vi "niRFUtil WFM Remove Frequency Offset - Fine.vi"(0 "Waveform In":T2 {"y" format="%.2f"; "dx" format="%^.2e"; "x0" format="%^.2e"}, 5 "Reference Waveform In":T2 {"y" format="%.2f"; "dx" format="%^.2e"; "x0" format="%^.2e"}, 7 "Filter Phase Estimates":T1=enum."True", 9 "Filter Length (samples)":i32=20) -> (4 "Waveform Out":T2 {"y" format="%.2f"; "dx" format="%^.2e"; "x0" format="%^.2e"}, 6 "Reference Waveform Out":T2 {"y" format="%.2f"; "dx" format="%^.2e"; "x0" format="%^.2e"}, 13 "Offset, Hz":sgl format="%^.2e")   [LabVIEW 2015, in "niRFUtil.lvlib"]
doc: "(c) Copyright 2006, National Instruments, Inc. This VI may not be duplicated, sold, or distributed without written consent from National Instruments."
uses:
  niRFUtil.lvlib
  Includes/niRFUtil INC Complex Waveform.ctl
  Includes/niRFUtil INC Complex Array.ctl
  Includes/niRFUtil INC Filter Phase Estimates.ctl
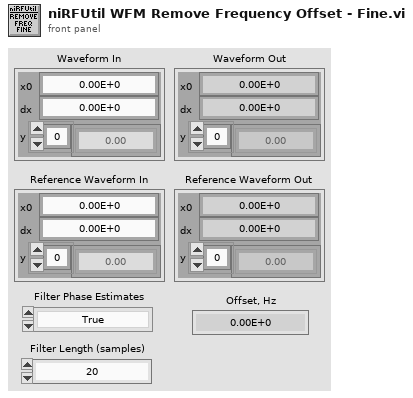
[diagram p1: front panel]
types:
  T1 = typedef "niRFUtil.lvlib/niRFUtil INC Filter Phase Estimates.ctl" = enum16{"False", "True"}
  T2 = typedef "niRFUtil.lvlib/niRFUtil INC Complex Waveform.ctl" = cluster{"x0":dbl, "dx":dbl, "y":T3}
  T3 = typedef "niRFUtil.lvlib/niRFUtil INC Complex Array.ctl" = csg[]
  T4 = typedef "niRFUtil.lvlib/niRFUtil INC Real Array.ctl" = sgl[]
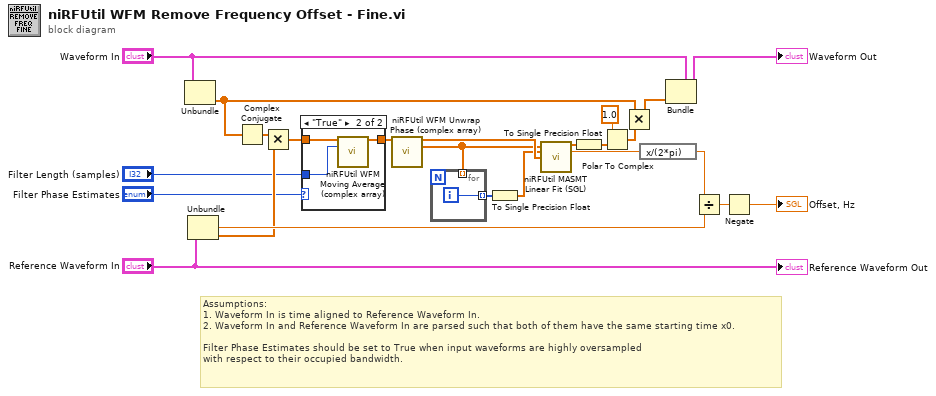
[diagram p0: block diagram]
diagram:
  # "Assumptions:\n1. Waveform In is time aligned to Reference Waveform In.\n2. Waveform In and Reference Waveform In are parsed such that both of them have the same starting time x0.\n\nFilter Phase Estimates should be set to True when input waveforms are highly oversampled\nwith respect to their occupied bandwidth."
  n1 = Unbundle("Waveform In") -> ("y"=w14:T3)  [unwired: 2 out]
  n2 = Unbundle("Reference Waveform In") -> ("dx"=w21:dbl, "y"=w20:T3)  [unwired: 1 out]
  n3 = Complex Conjugate(1:w14) -> (0:w23:T3)
  n4 = Multiply(x=w23, y=w20) -> (x*y=w24:T3)
  n5 = case shown="\"True\"" "Filter Phase Estimates" {
    tunnel: w24 -> [w25 w28]
    tunnel: [w25 w27] -> w4
    tunnel: "Filter Length (samples)" -> [_ w26]
    frame "False" {
    }
    frame "True" {
      n6 = call "niRFUtil WFM Moving Average (complex array).vi"("Array In"=w28, "Averaging Window (samples)"=w26) -> ("Averaged Array Out"=w27:T3)  [unwired: 13 in]
    }
  }
  n7 = call "niRFUtil WFM Unwrap Phase (complex array).vi"("Complex Vectors"=w4) -> ("Magnitude"=w8:T4, "Unwrapped Phase (rad)"=w3:T4)  [unwired: 13 in]
  n8 = for {
    tunnel: [w29] -> w7 mode=indexing
    tunnel: w3 -> [_] mode=indexing
    i -> [w29]
  }
  n9 = To Single Precision Float(number=w7) -> (single precision float=w6:sgl[])
  n10 = call "niRFUtil MASMT Linear Fit (SGL).vi"("Y"=w3, "X"=w6, "Weight"=w8) -> ("Best Linear Fit"=w12:sgl[], "slope"=w17:sgl)  [unwired: 8 in, 3 out]
  n11 = To Single Precision Float(number=w12) -> (single precision float=w5:sgl[])
  n12 = Polar To Complex(1:w5, 2:sgl 1.0) -> (0:w10:csg[])
  n13 = Multiply(x=w14, y=w10) -> (x*y=w13:T3)
  n14 = expression code="x/(2*pi)"(w17) -> (w19:sgl)
  n15 = Bundle(cluster="Waveform In", "y"=w13) -> (→"Waveform Out":T2)  [unwired: 2 out]
  n16 = Divide(x=w19, y=w21) -> (x/y=w22:dbl)
  n17 = Negate(x=w22) -> (-x=→"Offset, Hz":dbl)
  "Reference Waveform Out" <- "Reference Waveform In"
